vi "RT Driver VI.vi"(7 "Operation":T1, 11 "Device Reference in":T2 format="%.0x") -> (0 "Error Code":i32)   [LabVIEW 2015, in "SLSC EDS Engine.lvlib"]
uses:
  SLSC EDS Engine.lvlib
  <vilib>/NI Veristand/Custom Device API/Custom Device Item Ref.ctl
  <vilib>/NI Veristand/Custom Device API/Hardware Interface Driver VI Operation.ctl
  Shared/Compiled.Settings
  Shared/SLSC Static Settings.ctl
  SLSC CD API/SLSC CD Engine/SLSC Dynamic Channel.ctl
  SLSC CD API/SLSC CD Engine/SLSC Datatype.ctl
  Types/RTStateVariables.ctl
  <vilib>/NI/NIVS Inline Async API/_VS Inline Async API/VS Inline Async API/VS Inline Async API.lvclass
  <vilib>/NI/NIVS Inline Async API/_VS Inline Async API/VS Inline Async API/VS Inline Async API.lvclass/VS Inline Async API.ctl
  <vilib>/NI/NIVS Inline Async API/_Data Access Engine/Data Access Engine/Data Access Engine.lvclass/Data Access Engine.ctl
  <vilib>/NI/NIVS Inline Async API/_Data Access Engine/Access Type Classes/Write/Write.lvclass/Write.ctl
  <vilib>/NI/NIVS Inline Async API/_Data Access Engine/Access Type Classes/ReadWrite/ReadWrite.lvclass/ReadWrite.ctl
  <vilib>/NI/NIVS Inline Async API/_Data Access Engine/Access Type Classes/Read/Read.lvclass/Read.ctl
  <vilib>/NI/NIVS Inline Async API/_Data Access Engine/Data Access Engine/Methods/Data.Engine.Read Data from HW.vi
  <vilib>/NI/NIVS Inline Async API/_VS Inline Async API/Error Handling Process/SubVIs/Error.GetError.vi
  <vilib>/NI/NIVS Inline Async API/_Data Access Engine/Data Access Engine/Methods/Data.Engine.Write Data to HW.vi
  <vilib>/NI/NIVS Inline Async API/_Data Access Engine/Access Type Classes/ReadWrite/ReadWrite.EngineData.vi
  <vilib>/NI/NIVS Inline Async API/_Data Access Engine/Access Type Classes/Write/Write.EngineData.vi
  <vilib>/NI/NIVS Inline Async API/_Data Access Engine/Access Type Classes/Read/Read.EngineData.vi
  <vilib>/NI Veristand/Custom Device API/NI VeriStand - Get Channel Value by Data Reference.vi
  <vilib>/NI Veristand/Custom Device API/NI VeriStand - Set Channel Value by Data Reference.vi
  <vilib>/NI Veristand/Custom Device API/NI VeriStand - Get Channel Values by Block Data Reference.vi
  Shared/Constants.vi
  <vilib>/NI Veristand/Custom Device API/Get Item Property (Variant).vi
  <vilib>/NI Veristand/Custom Device API/Global Data Refs.vi
  <vilib>/NI VeriStand/Custom Device API/Custom Device API.lvlib
  Shared/SLSC EDS Shared.lvlib
  <vilib>/NI VeriStand/Custom Device Tools/Custom Device Utility Library/Custom Device Utility Library.lvlib
  SLSC CD API/SLSC CD Shared/SLSC CD Shared.lvlib
  SLSC CD API/SLSC CD Engine/SLSC CD Engine.lvlib
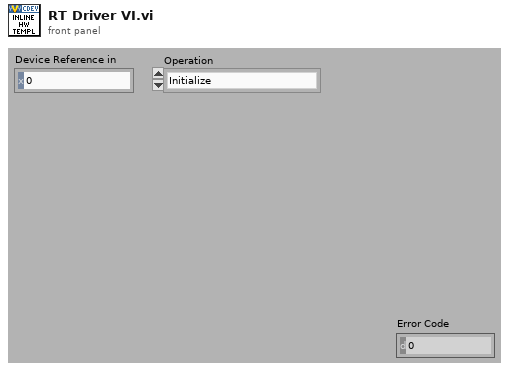
[diagram p1: front panel]
types:
  T1 = typedef "Custom Device API.lvlib/Hardware Interface Driver VI Operation.ctl" = enum16{"Initialize", "Start", "Read Data from HW", "Write Data to HW", "Close"}
  T2 = typedef "Custom Device API.lvlib/Custom Device Item Ref.ctl" = u64
  T3 = typedef "SLSC EDS Engine.lvlib/RTStateVariables.ctl" = cluster{"Async":refnum<class "VS Inline Async API.lvclass">, "Settings":T4}
  T4 = typedef "SLSC EDS Shared.lvlib/Compiled.Settings" = cluster{"Name":string, "SLSC Name or IP Address":string, "Slot #":i32, "Configuration Data":T5, "SLSC Get/Read Properties":T6[], "SLSC Set/Write Properties":T6[], "SLSC Dynamic Commands":T6[], "Support Modules":cluster{"Dev.ProductNumber":u32, "Dev.VendorNumber":u32}[]}
  T5 = typedef "SLSC EDS Shared.lvlib/SLSC Static Settings.ctl" = cluster{"Properties":cluster{"Boolean Properties":cluster{"property":refnum<k21>, "Value":bool, "SLSC Item":refnum<k21>, "reset value":bool}[], "Double Properties":cluster{"property":refnum<k21>, "Double Write":dbl, "SLSC Item":refnum<k21>, "Double Reset Value":dbl}[], "I32 Properties":cluster{"property":refnum<k21>, "Int32 Write":i32, "SLSC Item":refnum<k21>, "Int32 Reset Value":i32}[], "I64 Properties":cluster{"property":refnum<k21>, "Int64 Write":i64, "SLSC Item":refnum<k21>, "Int64 Reset Value":i64}[], "String Properties":cluster{"property":refnum<k21>, "String Write":string, "SLSC Item":refnum<k21>, "String Reset Value":string}[], "U32 Properties":cluster{"property":refnum<k21>, "UInt32 Write":u32, "SLSC Item":refnum<k21>, "UInt32 Reset Value":u32}[], "U64 Properties":cluster{"property":refnum<k21>, "UInt64 Write":u64, "SLSC Item":refnum<k21>, "UInt64 Reset Value":u64}[]}, "Commands":T6[], "Reset Commands":T6[], "Apply Values on Deployment":bool, "Apply Reset on Undeployment":bool}
  T6 = typedef "SLSC CD Shared.lvlib/SLSC Dynamic Channel.ctl" = cluster{"SLSC Item":string, "property":string, "Data Type":T7}
  T7 = typedef "SLSC CD Shared.lvlib/SLSC Datatype.ctl" = enum16{"Bool", "Double", "I32", "I64", "String", "U32", "U64"}
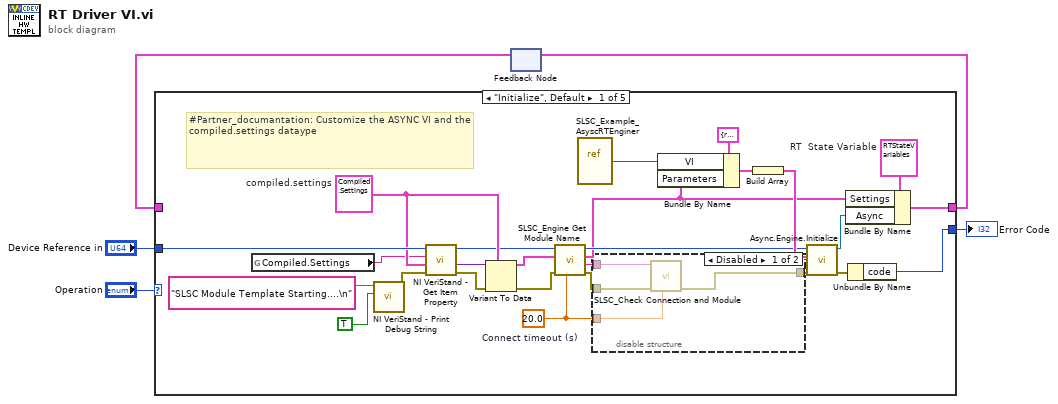
[diagram p0: block diagram]
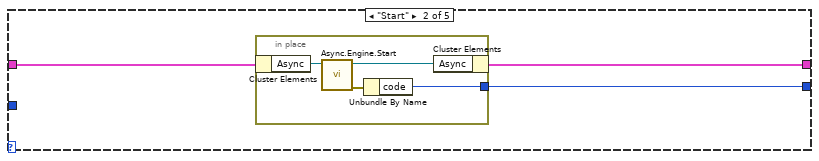
[diagram p3: hidden frame]
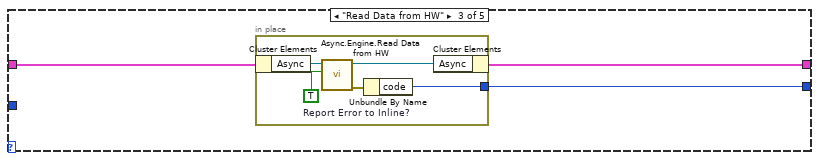
[diagram p4: hidden frame]
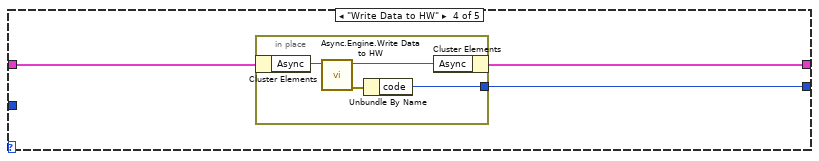
[diagram p5: hidden frame]
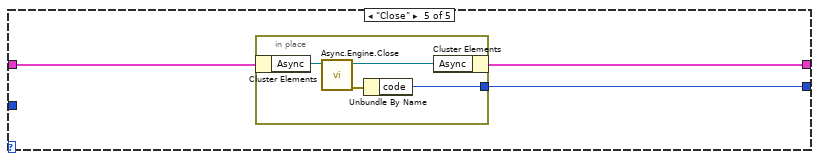
[diagram p6: hidden frame]
diagram:
  n1 = feedback #1() -> (w3:T3)  [unwired: 1 out]
  n2 = case shown="\"Initialize\", Default" "Operation" {
    tunnel: [w29 w38 w44 w52 w60] -> w4
    tunnel: w3 -> [_ w39 w46 w53 w61]
    tunnel: "Device Reference in" -> [w26 _ _ _ _]
    tunnel: [w31 w37 w45 w54 w59] -> w1
    frame "Initialize", Default {
      w8 = 20.0  # Connect timeout (s)
      w21 = T3 {"Async"=refnum, "Settings"={"Name"="", "SLSC Name or IP Address"="", "Slot #"=0, "Configuration Data"={"Properties"={"Boolean Properties"=[], "Double Properties"=[], "I32 Properties"=[], "I64 Properties"=[], "String Properties"=[], "U32 Properties"=[], "U64 Properties"=[]}, "Commands"=[], "Reset Commands"=[], "Apply Values on Deployment"=TRUE, "Apply Reset on Undeployment"=TRUE}, "SLSC Get/Read Properties"=[], "SLSC Set/Write Properties"=[], "SLSC Dynamic Commands"=[], "Support Modules"=[]}}  # RT  State Variable
      w22 = T4 {"Name"="", "SLSC Name or IP Address"="", "Slot #"=0, "Configuration Data"={"Properties"={"Boolean Properties"=[], "Double Properties"=[], "I32 Properties"=[], "I64 Properties"=[], "String Properties"=[], "U32 Properties"=[], "U64 Properties"=[]}, "Commands"=[], "Reset Commands"=[], "Apply Values on Deployment"=TRUE, "Apply Reset on Undeployment"=TRUE}, "SLSC Get/Read Properties"=[], "SLSC Set/Write Properties"=[], "SLSC Dynamic Commands"=[], "Support Modules"=[]}  # compiled.settings
      # "#Partner_documantation: Customize the ASYNC VI and the compiled.settings dataype"
      n3 = global read "Constants.vi" "Compiled.Settings"() -> (w17:string)
      n4 = call <vilib>:"NI VeriStand - Print Debug String.vi"("Add to log file? (T)"=TRUE, "Message"="SLSC Module Template Starting....\n") -> ("error out"=w19:errorcluster)  [unwired: 9 in]
      n5 = call-poly <vilib>:"NI VeriStand - Get Item Property.vi"("error in (no error)"=w19, "Default Value"=w22, "Property Name"=w17, "Item Ref in"=w26) -> ("error out"=w25:errorcluster, "Value"=w24:variant, "Item Ref out"=w13:T2)  [unwired: 4 in, 1 out]
      n6 = Variant To Data(error in=w25, type=w22, Variant=w24) -> (data=w12:T4, error out=w10:errorcluster)
      n7 = call "SLSC_Engine Get Module Name.vi"("Connect timeout (s)"=w8, "error in (no error)"=w10, "compiled.settings"=w12, "Item Ref in"=w13) -> ("error out"=w9:errorcluster, "SLSC Module Name"=w6:string, "compiled.settings out"=w7:T4, "Item Ref out"=w11:T2)  [unwired: 4 in]
      n8 = vi-ref "SLSC_Example_AsyscRTEnginer.vi"() -> (w15:refnum<vi>)
      n9 = disable-structure shown="Disabled" {
        disable-tunnel: [w35 w36] -> w14
        disable-tunnel: w9 -> [w34 w36]
        disable-tunnel: w8 -> [w33 _]
        disable-tunnel: w6 -> [w32 _]
        frame Disabled {
          n10 = call "SLSC_Check Connection and Module.vi"("Connect timeout (s)"=w33, "error in (no error)"=w34, "devices"=w32) -> ("error out"=w35:errorcluster)  [unwired: 7 in, 1 out]
        }
        frame Enabled {
        }
      }
      n11 = Bundle By Name(cluster=cluster{"VI":refnum<vi>, "Parameters":variant} {"VI"=refnum, "Parameters"=variant} ("Process"), "VI"=w15, "Parameters"=w7) -> (w27:cluster{"VI":refnum<vi>, "Parameters":variant})
      n12 = Build Array(w27) -> (w20:cluster{"VI":refnum<vi>, "Parameters":variant}[])
      n13 = call <vilib>:"Async.Engine.Initialize.vi"("error in (no error)"=w14, "Processes"=w20, "Custom Device Ref"=w11) -> ("error out"=w23:errorcluster, "Async"=w30:refnum<class "VS Inline Async API.lvclass">)  [unwired: 7 in]
      n14 = Bundle By Name(cluster=w21, "Settings"=w7, "Async"=w30) -> (w29:T3)
      n15 = Unbundle By Name(w23) -> ("code"=w31:i32)
    }
    frame "Start" {
      n16 = in-place {
        in-place-border: [w40] -> w37
        n17 = in-place-cluster #2(w39) -> ("Async"=w43:refnum<class "VS Inline Async API.lvclass">)
        n18 = call <vilib>:"Async.Engine.Start.vi"("VS Inline Async API in"=w43) -> ("error out"=w41:errorcluster, "VS Inline Async API out"=w42:refnum<class "VS Inline Async API.lvclass">)  [unwired: 9 in]
        n19 = Unbundle By Name(w41) -> ("code"=w40:i32)
        n20 = in-place-cluster #2("Async"=w42) -> (w38:T3)
      }
    }
    frame "Read Data from HW" {
      n21 = in-place {
        in-place-border: [w49] -> w45
        w47 = TRUE  # Report Error to Inline?
        n22 = in-place-cluster #3(w46) -> ("Async"=w51:refnum<class "VS Inline Async API.lvclass">)
        n23 = call <vilib>:"Async.Engine.Read Data from HW.vi"("Report Error to Inline?"=w47, "Async in"=w51) -> ("error out"=w48:errorcluster, "Async out"=w50:refnum<class "VS Inline Async API.lvclass">)  [unwired: 8 in]
        n24 = Unbundle By Name(w48) -> ("code"=w49:i32)
        n25 = in-place-cluster #3("Async"=w50) -> (w44:T3)
      }
    }
    frame "Write Data to HW" {
      n26 = in-place {
        in-place-border: [w58] -> w54
        n27 = in-place-cluster #4(w53) -> ("Async"=w56:refnum<class "VS Inline Async API.lvclass">)
        n28 = call <vilib>:"Async.Engine.Write Data to HW.vi"("VS Inline Async API in"=w56) -> ("error out"=w57:errorcluster, "VS Inline Async API out"=w55:refnum<class "VS Inline Async API.lvclass">)  [unwired: 9 in]
        n29 = Unbundle By Name(w57) -> ("code"=w58:i32)
        n30 = in-place-cluster #4("Async"=w55) -> (w52:T3)
      }
    }
    frame "Close" {
      n31 = in-place {
        in-place-border: [w63] -> w59
        n32 = in-place-cluster #5(w61) -> ("Async"=w65:refnum<class "VS Inline Async API.lvclass">)
        n33 = call <vilib>:"Async.Engine.Close.vi"("Async in"=w65) -> ("error out"=w62:errorcluster, "Async out"=w64:refnum<class "VS Inline Async API.lvclass">)  [unwired: 9 in]
        n34 = Unbundle By Name(w62) -> ("code"=w63:i32)
        n35 = in-place-cluster #5("Async"=w64) -> (w60:T3)
      }
    }
  }
  "Error Code" <- w1
  n36 = feedback-in #1(w4) -> ()
